vi "FTW-Endpoint-TCP-Request-Worker.vi"(0 "TCP Endpoint":refnum<class "FTW-Endpoint-TCP.lvclass">, 5 "Address":string) -> ()   [LabVIEW 2013, in "FTW-Endpoint-TCP.lvclass"]
uses:
  FTW-Endpoint-TCP.lvclass
  FTW-Endpoint-TCP.lvclass/FTW-Endpoint-TCP.ctl
  Payload/FTW-MessagePayload.ctl
panel:
  out "connected":bool
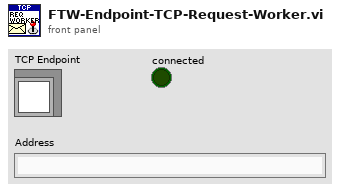
[diagram p1: front panel]
types:
  T1 = typedef "FTW-MessagePayload.ctl" = cluster{"Header":string, "Body":string, "FTW: Sender Identity":string, "FTW: Reply Address":string, "FTW: Reply Error":errorcluster}
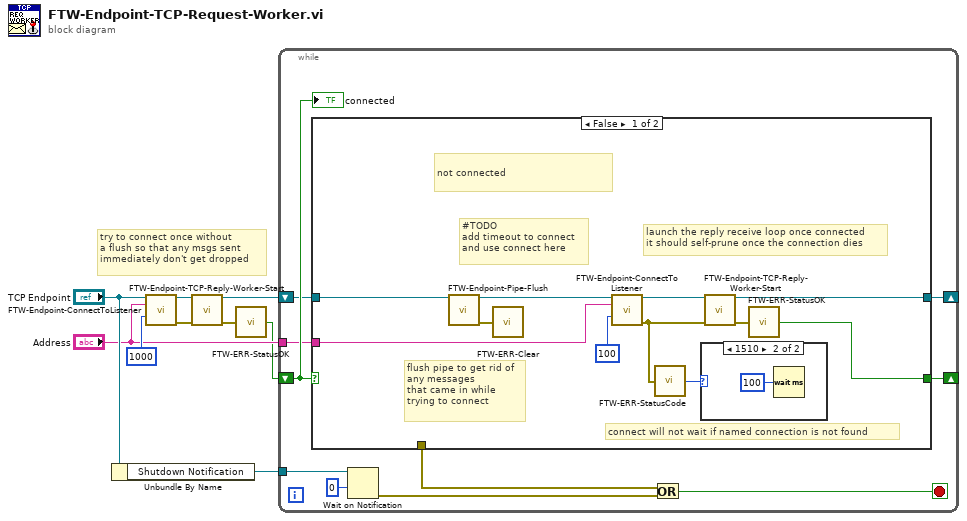
[diagram p0: block diagram]
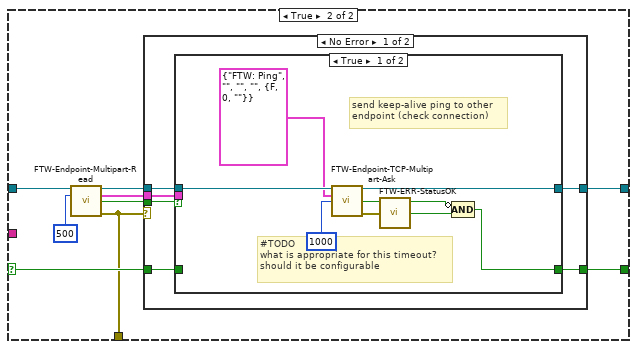
[diagram p3: hidden frame]
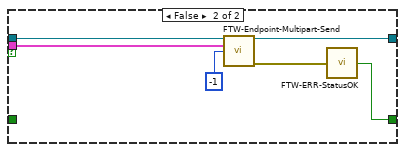
[diagram p4: hidden frame]
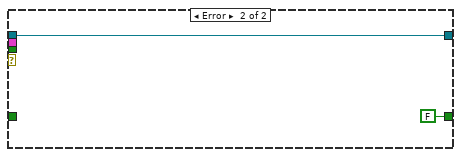
[diagram p5: hidden frame]
diagram:
  # "try to connect once without\na flush so that any msgs sent\nimmediately don't get dropped"
  n1 = Unbundle By Name("TCP Endpoint") -> ("Shutdown Notification"=w9:refnum<notifier>)
  n2 = call-dynamic "FTW-Endpoint-ConnectToListener.vi"("FTW-Endpoint In"="TCP Endpoint", "Address"="Address", "Timeout"=1000) -> ("FTW-Endpoint Out"=w6:refnum<class "FTW-Endpoint-TCP.lvclass">, "error out"=w5:errorcluster)  [unwired: 10 in, 1 out]
  n3 = call-dynamic "FTW-Endpoint-TCP-Reply-Worker-Start.vi"("FTW-Endpoint-TCP In"=w6, "error in"=w5) -> ("FTW-Endpoint-TCP Out"=w3:refnum<class "FTW-Endpoint-TCP.lvclass">, "error out"=w8:errorcluster)  [unwired: 12 in]
  n4 = call "FTW-ERR-StatusOK.vi"("error to check"=w8) -> ("Status OK?"=w1:bool)
  n5 = while {
    shift-right: [w16] -> _
    shift-left: w1 -> [w19]
    shift-right: [w17] -> _
    shift-left: w3 -> [w12]
    tunnel: "Address" -> [w18]
    tunnel: w9 -> [w14]
    stop <- w11 stop-if-true
    n6 = case shown="False" w19 {
      selector: w19 -> [_ w37]
      tunnel: w18 -> [w30 _]
      tunnel: [w25 w39] -> w17
      tunnel: [w29 w38] -> w16
      tunnel: w12 -> [w27 w40]
      tunnel: [_ w35] -> w10
      frame False {
        # "connect will not wait if named connection is not found"
        # "flush pipe to get rid of\nany messages\nthat came in while\ntrying to connect"
        # "launch the reply receive loop once connected\nit should self-prune once the connection dies"
        # "not connected"
        # "#TODO\nadd timeout to connect\nand use connect here"
        n7 = call-dynamic "FTW-Endpoint-Pipe-Flush.vi"("FTW Endpoint"=w27) -> ("FTW Endpoint out"=w24:refnum<class "FTW-Endpoint-TCP.lvclass">, "error out"=w23:errorcluster)  [unwired: 13 in]
        n8 = call "FTW-ERR-Clear.vi"("error to snuff"=w23) -> ()  [unwired: 1 out]
        n9 = call-dynamic "FTW-Endpoint-ConnectToListener.vi"("FTW-Endpoint In"=w24, "Address"=w30, "Timeout"=100) -> ("FTW-Endpoint Out"=w22:refnum<class "FTW-Endpoint-TCP.lvclass">, "error out"=w21:errorcluster)  [unwired: 10 in, 1 out]
        n10 = call "FTW-ERR-StatusCode.vi"("error to check"=w21) -> ("Code"=w20:i32)
        n11 = case shown="1510" w20 {
          frame 0, Default {
          }
          frame 1510 {
            n12 = Wait (ms)(milliseconds to wait=u32 100) -> ()  [unwired: 1 out]
          }
        }
        n13 = call-dynamic "FTW-Endpoint-TCP-Reply-Worker-Start.vi"("FTW-Endpoint-TCP In"=w22, "error in"=w21) -> ("FTW-Endpoint-TCP Out"=w25:refnum<class "FTW-Endpoint-TCP.lvclass">, "error out"=w26:errorcluster)  [unwired: 12 in]
        n14 = call "FTW-ERR-StatusOK.vi"("error to check"=w26) -> ("Status OK?"=w29:bool)
      }
      frame True {
        n15 = call-dynamic "FTW-Endpoint-Multipart-Read.vi"("FTW Endpoint"=w40, "Timeout"=500) -> ("FTW Endpoint out"=w36:refnum<class "FTW-Endpoint-TCP.lvclass">, "Message Received"=w32:T1, "Timed out?"=w33:bool, "error out"=w35:errorcluster)  [unwired: 10 in]
        n16 = case shown="No Error" w35 {
          tunnel: [w46 w62] -> w39
          tunnel: [w45 FALSE ("Status OK?")] -> w38
          tunnel: w37 -> [w44 _]
          tunnel: w36 -> [w43 w62]
          tunnel: w33 -> [w42 _]
          tunnel: w32 -> [w41 _]
          frame No Error {
            n17 = case shown="True" w42 {
              tunnel: w43 -> [w54 w60]
              tunnel: [w53 w59] -> w46
              tunnel: [w49 w57] -> w45
              tunnel: w44 -> [_ _]
              tunnel: w41 -> [_ w55]
              frame True {
                # "send keep-alive ping to other\nendpoint (check connection)"
                # "#TODO\nwhat is appropriate for this timeout?\nshould it be configurable"
                n18 = call-dynamic "FTW-Endpoint-TCP-Multipart-Ask.vi"("FTW Endpoint"=w54, "Message"=T1 {"Header"="FTW: Ping", "Body"="", "FTW: Sender Identity"="", "FTW: Reply Address"="", "FTW: Reply Error"={"status"=FALSE, "code"=0, "source"=""}}, "Read Timeout"=1000) -> ("FTW Endpoint out"=w53:refnum<class "FTW-Endpoint-TCP.lvclass">, "Read Timed out?"=w48:bool, "error out"=w52:errorcluster)  [unwired: 8 in, 2 out]
                n19 = call "FTW-ERR-StatusOK.vi"("error to check"=w52) -> ("Status OK?"=w51:bool)
                n20 = Compound Arithmetic op=AND(invert w48, w51) -> (w49:bool)
              }
              frame False {
                n21 = call-dynamic "FTW-Endpoint-Multipart-Send.vi"("FTW Endpoint"=w60, "Message"=w55, "Timeout"=-1) -> ("FTW Endpoint out"=w59:refnum<class "FTW-Endpoint-TCP.lvclass">, "error out"=w58:errorcluster)  [unwired: 10 in, 1 out]
                n22 = call "FTW-ERR-StatusOK.vi"("error to check"=w58) -> ("Status OK?"=w57:bool)
              }
            }
          }
          frame Error {
          }
        }
      }
    }
    n23 = Wait on Notification(notifier=w14, timeout in ms (-1)=0) -> (error out=w13:errorcluster)  [unwired: 2 in, 3 out]
    n24 = Or(x=w10, y=w13) -> (x .or. y?=w11:bool)
    "connected" <- w19
  }
